vi "Motion@Home__Parameter.vi"(1 "ParamterIn":string) -> (0 "ParamterOut":string)   [LabVIEW 2019]
panel:
  in  "AXIS":string(combo)="X"
  in  "Mode":string(combo)
  in  "MotorSelect":string(combo)
  in  "Confirm":bool
  # "Motor@Home $Motor,$AXIS(,CounterOnly)"
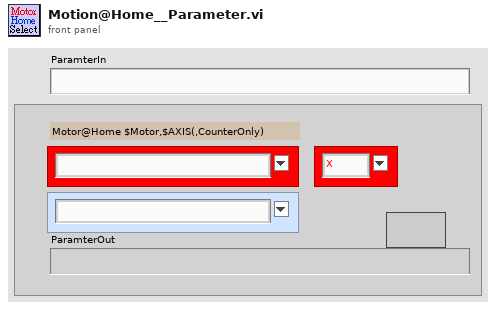
[diagram p1: front panel]
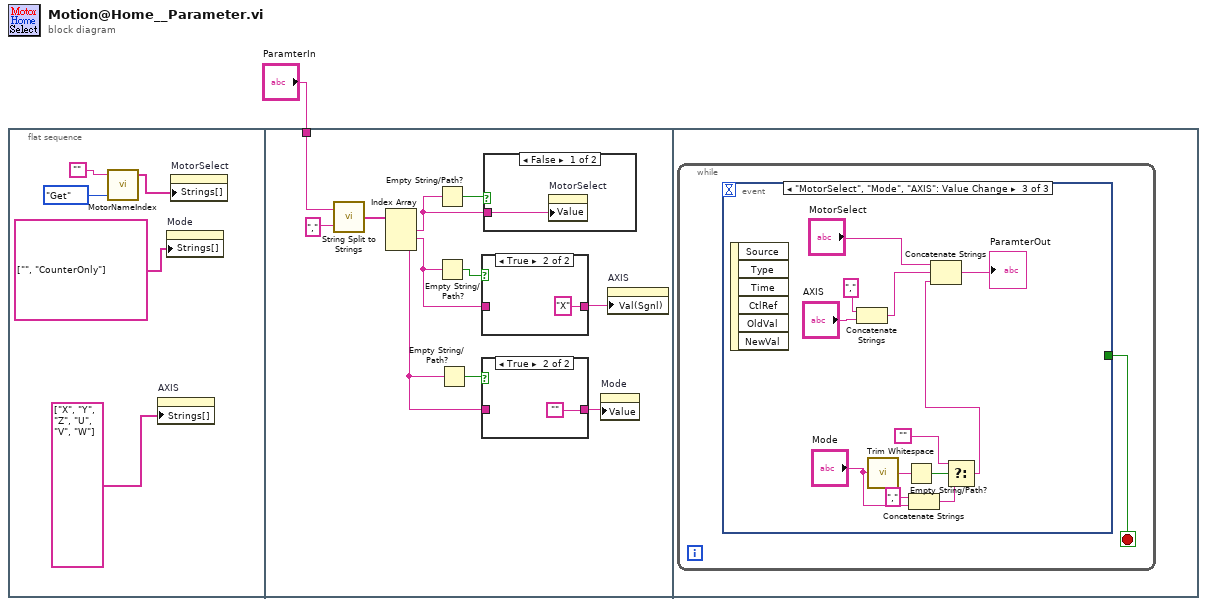
[diagram p0: block diagram]
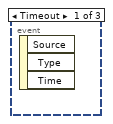
[diagram p5: hidden frame]
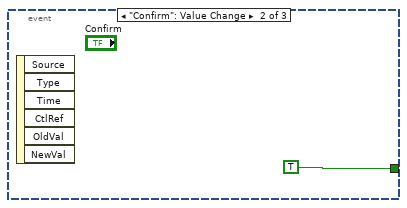
[diagram p6: hidden frame]
diagram:
  n1 = flat-sequence {
    tunnel: "ParamterIn" -> [w15]
    frame #0 {
      n2 = call "MotorNameIndex.vi"("OP"=enum16{"Get", "Update", "Init"}."Get", "MotorName"="") -> ("MotorList"=w3:string[])  [unwired: 1 in, 2 out]
      n3 = property on="AXIS" class="CmbBox"("Strings[]"=string[] ["X", "Y", "Z", "U", "V", "W"] ("Strings []")) -> ()  [unwired: 2 in, 2 out]
      n4 = property on="Mode" class="CmbBox"("Strings[]"=string[] ["", "CounterOnly"] ("Strings []")) -> ()  [unwired: 2 in, 2 out]
      n5 = property on="MotorSelect" class="CmbBox"("Strings[]"=w3) -> ()  [unwired: 2 in, 2 out]
    }
    frame #1 {
      n6 = call "String Split to Strings.vi"("search string/char (-)"=",", "String"=w15) -> ("Array"=w17:string[])
      n7 = Index Array(array=w17) -> (element #1=w13:string, element #2=w11:string, element #3=w8:string)  [unwired: 3 in]
      n8 = Empty String/Path?(string/path=w13) -> (empty?=w14:bool)
      n9 = Empty String/Path?(string/path=w11) -> (empty?=w12:bool)
      n10 = Empty String/Path?(string/path=w8) -> (empty?=w9:bool)
      n11 = case shown="True" w12 {
        tunnel: [w20 "X"] -> w10
        tunnel: w11 -> [w20 _]
        frame False {
        }
        frame True {
        }
      }
      n12 = case shown="True" w9 {
        tunnel: w8 -> [w18 _]
        tunnel: [w18 ""] -> w7
        frame False {
        }
        frame True {
        }
      }
      n13 = case shown="False" w14 {
        tunnel: w13 -> [w22 _]
        frame False {
          n14 = property on="MotorSelect" class="CmbBox"("Value"=w22) -> ()  [unwired: 2 in, 2 out]
        }
        frame True {
        }
      }
      n15 = property on="Mode" class="CmbBox"("Value"=w7) -> ()  [unwired: 2 in, 2 out]
      n16 = property on="AXIS" class="CmbBox"("Val(Sgnl)"=w10) -> ()  [unwired: 2 in, 2 out]
    }
    frame #2 {
      n17 = while {
        stop <- w23 stop-if-true
        n18 = event shown="[2] \"MotorSelect\", \"Mode\", \"AXIS\": Value Change" {
          selector: _ -> [_ _ _]
          dyn-events: _ -> [_ _ _]
          timeout: _ -> [_ _ _]
          tunnel: [_ TRUE _] -> w23
          event Timeout {
            n19 = event-data() -> ()  [unwired: 1 in, 3 out]
          }
          event "Confirm": Value Change {
            n20 = event-data() -> ()  [unwired: 1 in, 6 out]
          }
          event "MotorSelect", "Mode", "AXIS": Value Change {
            n21 = event-data() -> ()  [unwired: 1 in, 6 out]
            n22 = Concatenate Strings("," ("string"), "AXIS") -> (w25:string)
            n23 = call <vilib>:"Trim Whitespace.vi"("string"="Mode") -> ("trimmed string"=w30:string)  [unwired: 1 in]
            n24 = Empty String/Path?(string/path=w30) -> (empty?=w31:bool)
            n25 = Concatenate Strings("," ("string"), "Mode") -> (w33:string)
            n26 = Select(t="", s=w31, f=w33) -> (s? t:f=w28:string)
            n27 = Concatenate Strings("MotorSelect", w25, w28) -> (→"ParamterOut":string)
          }
        }
      }
    }
  }
